vi "Write Goto.vi"(8 "error in (no error)":errorcluster, 9 "Enable warning? (T)":bool=TRUE, 10 "Target":dbl[unit], 11 "Power Supply in":refnum<class "Power Supply.lvclass">) -> (0 "error out":errorcluster, 3 "Power Supply out":refnum<class "Power Supply.lvclass">)   [LabVIEW 2009, in "Power Supply.lvclass"]
doc: "Tells magnet to now go to the target field (if Goto Zero is set to true, goes to 0 instead)."
uses:
  Power Supply.lvclass
  Power Supply.lvclass/Power Supply.ctl
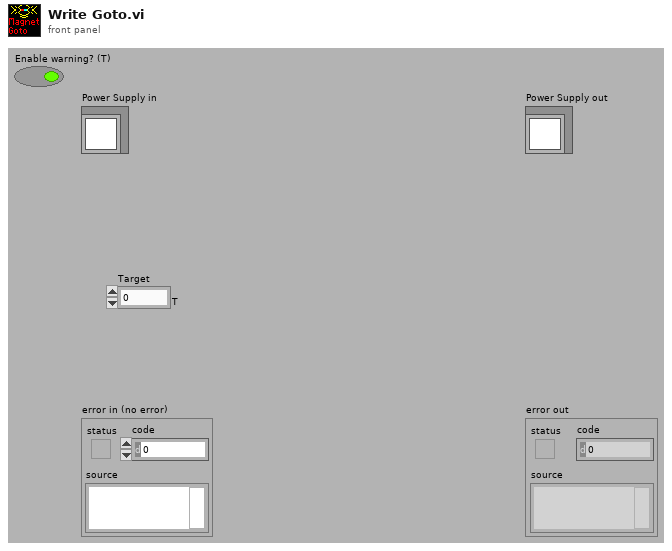
[diagram p1: front panel]
types:
  T1 = typedef "PSIO.ctl" = cluster{"Address":T2, "Version":enum16{"PS", "IPS"}}
  T2 = typedef "OxfordAddress.ctl" = cluster{"Com Port":i32, "ISOBUS Address":i32, "GPIB Address":i16, "Communication":enum16{"RS232", "ISOBUS", "GPIB", "Gateway"}}
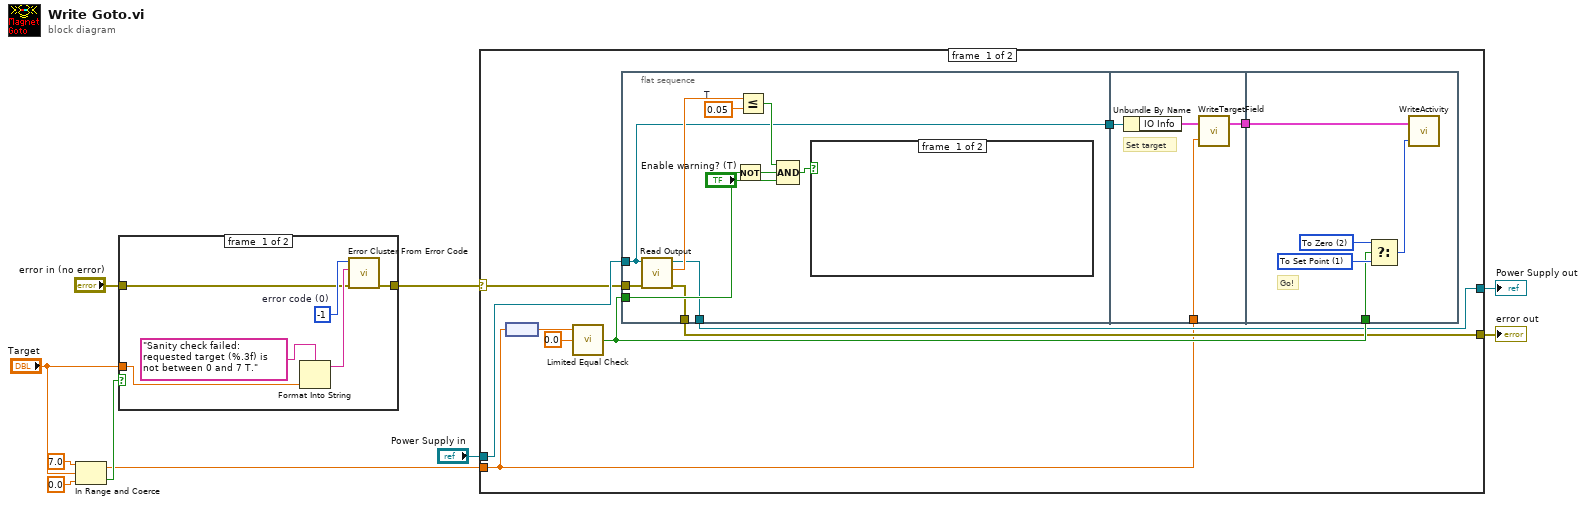
[diagram p0: block diagram]
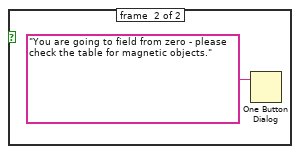
[diagram p3: hidden frame]
diagram:
  n1 = In Range and Coerce(upper limit=dbl[unit] 7.0, x="Target", lower limit=dbl[unit] 0.0) -> (coerced(x)=w1:dbl[unit], In Range?=w3:bool)
  n2 = case shown="False" w3 {
    tunnel: [w16 w17] -> w5
    tunnel: "error in (no error)" -> [w11 w17]
    tunnel: "Target" -> [w13 _]
    frame #0 {
      w15 = -1  # error code (0)
      n3 = Format Into String(format string="Sanity check failed: requested target (%.3f) is not between 0 and 7 T." ("error message (\"\")"), w13) -> (resulting string=w12:string)  [unwired: 2 in, 1 out]
      n4 = call <vilib>:"Error Cluster From Error Code.vi"("error in (no error)"=w11, "error message (\"\")"=w12, "error code (0)"=w15) -> ("error out"=w16:errorcluster)  [unwired: 6 in]
    }
    frame #1 {
    }
  }
  n5 = case shown="No Error" w5 {
    selector: w5 -> [w19 w49]
    tunnel: "Power Supply in" -> [w22 w50]
    tunnel: [w21 w50] -> w9
    tunnel: [w20 w49] -> w8
    tunnel: w1 -> [w18 _]
    frame #0 {
      n6 = node(w18) -> (w25:dbl)
      n7 = call "Limited Equal Check.vi"("number2"=0.0, "number1"=w25) -> ("equal?"=w23:bool)  [unwired: 1 in, 2 out]
      n8 = flat-sequence {
        tunnel: [w31] -> w27
        tunnel: w23 -> [w33]
        tunnel: w22 -> [w31]
        tunnel: [w32] -> w21
        tunnel: w19 -> [w30]
        tunnel: [w29] -> w20
        tunnel: [w43] -> w26
        tunnel: w27 -> [w42]
        tunnel: w18 -> [w40]
        tunnel: w26 -> [w48]
        tunnel: w23 -> [w44]
        frame #0 {
          w37 = dbl[unit] 0.05  # T
          n9 = call-dynamic "Read Output.vi"("error in (no error)"=w30, "Power Supply in"=w31) -> ("error out"=w29:errorcluster, "Field"=w38:dbl[unit], "Power Supply out"=w32:refnum<class "Power Supply.lvclass">)  [unwired: 6 in, 1 out]
          n10 = Not(x=w33) -> (.not. x?=w34:bool)
          n11 = Less Or Equal?(x=w38, y=w37) -> (x <= y?=w36:bool)
          n12 = Compound Arithmetic op=AND(w36, w34, "Enable warning? (T)") -> (w35:bool)
          n13 = case shown="True" w35 {
            frame #0 {
            }
            frame #1 {
              n14 = One Button Dialog(message="You are going to field from zero - please check the table for magnetic objects.") -> ()  [unwired: 2 out]
            }
          }
        }
        frame #1 {
          # "Set target"
          n15 = Unbundle By Name(w42) -> ("IO Info"=w41:T1)
          n16 = call "WriteTargetField.vi"("Target Field"=w40, "IO Info"=w41) -> ("IO Info"=w43:T1)  [unwired: 1 out]
        }
        frame #2 {
          w45 = u16 2 items=["Hold", "To Set Point", "To Zero", "Clamp"] ("Activity")
          w47 = u16 1 items=["Hold", "To Set Point", "To Zero", "Clamp"] ("Activity")
          # "Go!"
          n17 = Select(t=w45, s=w44, f=w47) -> (s? t:f=w46:u16)
          n18 = call "WriteActivity.vi"("Activity"=w46, "IO Info"=w48) -> ()  [unwired: 2 out]
        }
      }
    }
    frame #1 {
    }
  }
  "error out" <- w8
  "Power Supply out" <- w9
